vi "Path Apply Inkscape Ratio.vi"(1 "paths in":T2(array[cluster])) -> (0 "paths out":T2(array[cluster]))   [LabVIEW 2019]
uses:
  <vilib>/Analysis/Matrix/Datatypes/RealMatrix.ctl
  Global Variables.vi
  <vilib>/Analysis/Matrix/NI_Matrix.lvlib
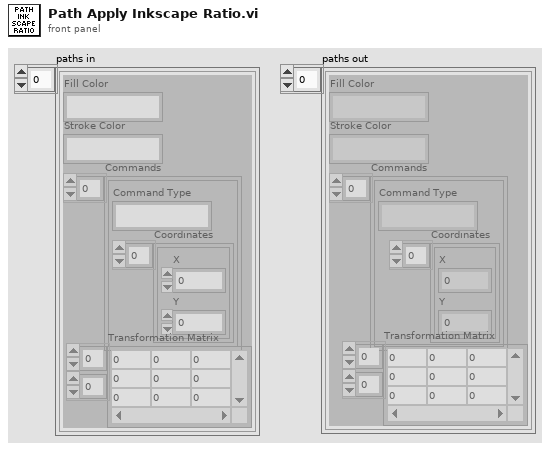
[diagram p1: front panel]
types:
  T1 = typedef "NI_Matrix.lvlib/RealMatrix.ctl" = dbl[][]
  T2 = cluster{"Fill Color":string, "Stroke Color":string, "Commands":cluster{"Command Type":string, "Coordinates":cluster{"X":dbl, "Y":dbl}[]}[], "Transformation Matrix":T1}[]
  T3 = cluster{"Command Type":string, "Coordinates":cluster{"X":dbl, "Y":dbl}[]}[]
  T4 = cluster{"Command Type":string, "Coordinates":cluster{"X":dbl, "Y":dbl}[]}
  T5 = cluster{"Fill Color":string, "Stroke Color":string, "Commands":cluster{"Command Type":string, "Coordinates":cluster{"X":dbl, "Y":dbl}[]}[], "Transformation Matrix":T1}
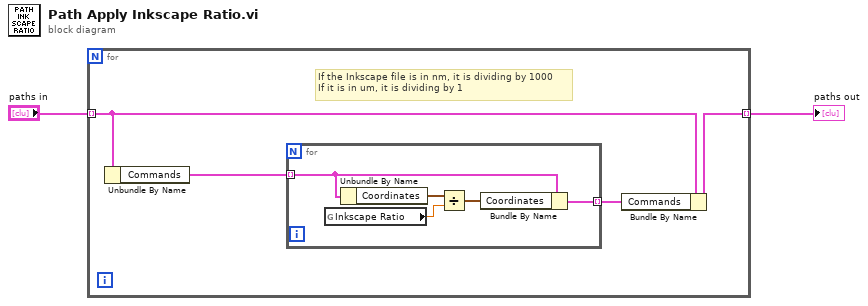
[diagram p0: block diagram]
diagram:
  n1 = for {
    tunnel: "paths in" -> [w4] mode=indexing
    tunnel: [w3] -> w2 mode=indexing
    # "If the Inkscape file is in nm, it is dividing by 1000\nIf it is in um, it is dividing by 1"
    n2 = Unbundle By Name(w4) -> ("Commands"=w6:T3)
    n3 = for {
      tunnel: w6 -> [w9] mode=indexing
      tunnel: [w8] -> w5 mode=indexing
      n4 = global read "Global Variables.vi" "Inkscape Ratio"() -> (w7:dbl)
      n5 = Unbundle By Name(w9) -> ("Coordinates"=w11:cluster{"X":dbl, "Y":dbl}[])
      n6 = Divide(x=w11, y=w7) -> (x/y=w10:cluster{"X":dbl, "Y":dbl}[])
      n7 = Bundle By Name(cluster=w9, "Coordinates"=w10) -> (w8:T4)
    }
    n8 = Bundle By Name(cluster=w4, "Commands"=w5) -> (w3:T5)
  }
  "paths out" <- w2
